vi "presentation_software.vi"() -> ()   [LabVIEW 2014]
uses:
  stateCtl.ctl
  <vilib>/Instr/_visa.llb/VISA Configure Serial Port (Instr).vi
panel:
  out "String":string
  in  "AnalogOutputDT":dbl(slide) scale=0.0..100.0
  out "Led1":bool
  in  "Output1":bool
  out "Led0":bool
  in  "Output0":bool
  out "S6":dbl
  out "S5":dbl
  out "S4":dbl
  out "S3":dbl
  out "S2":dbl
  out "S1":dbl
  out "S0":dbl
  in  "Tab Control":T1(tab)
  out "Frequency":dbl(graph)
  out "Temperature 1":dbl(graph)
  out "Temperature 2":dbl(graph)
  out "Load Cell 1":dbl(graph)
  out "Load Cell 2":dbl(graph)
  out "Vibration":dbl(graph)
  out "Analog Output":dbl(graph)
  out "exitLed":bool
  out "statusBar":string="     "
  in  "startButton":bool
  out "stopLed":bool
  out "startLed":bool
  in  "VISA Serial Port":refnum<visa-resource-name>
  in  "exitButton":bool
  in  "stopButton":bool
  out "FE":string
  out "FP":string
  out "isRunning":bool
  out "state":T2=enum."exit"
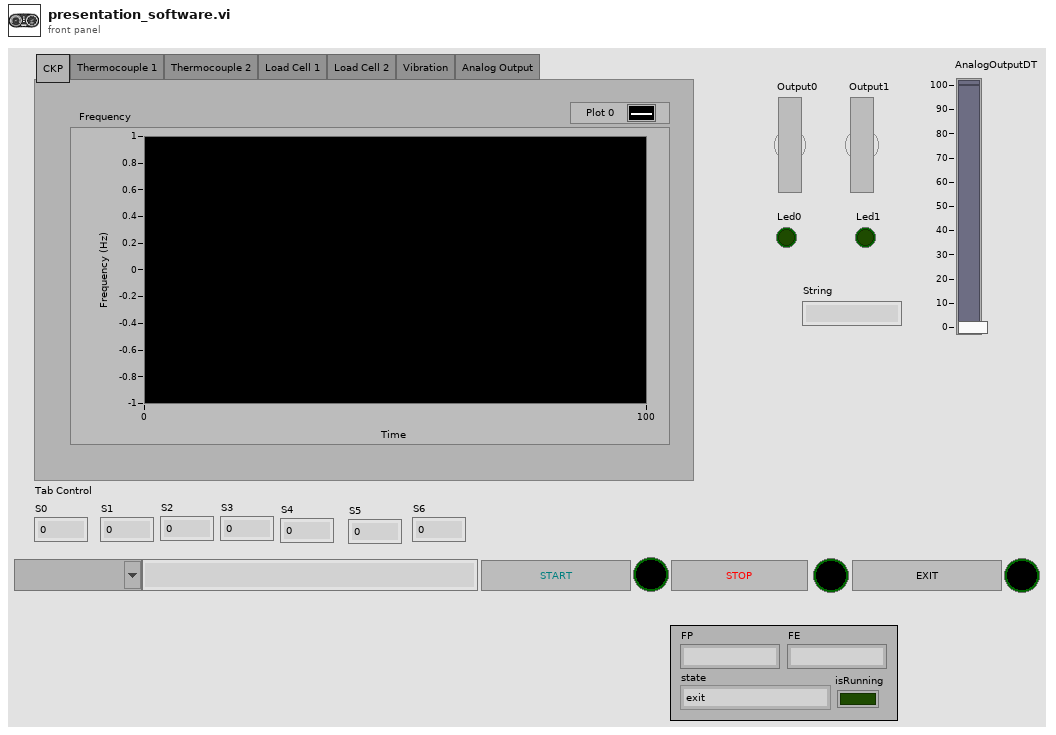
[diagram p1: front panel]
types:
  T1 = enum32{"CKP", "Thermocouple 1", "Thermocouple 2", "Load Cell 1", "Load Cell 2", "Vibration", "Analog Output"}
  T2 = typedef "stateCtl.ctl" = enum16{"init", "ready", "running", "stopped", "exit"}
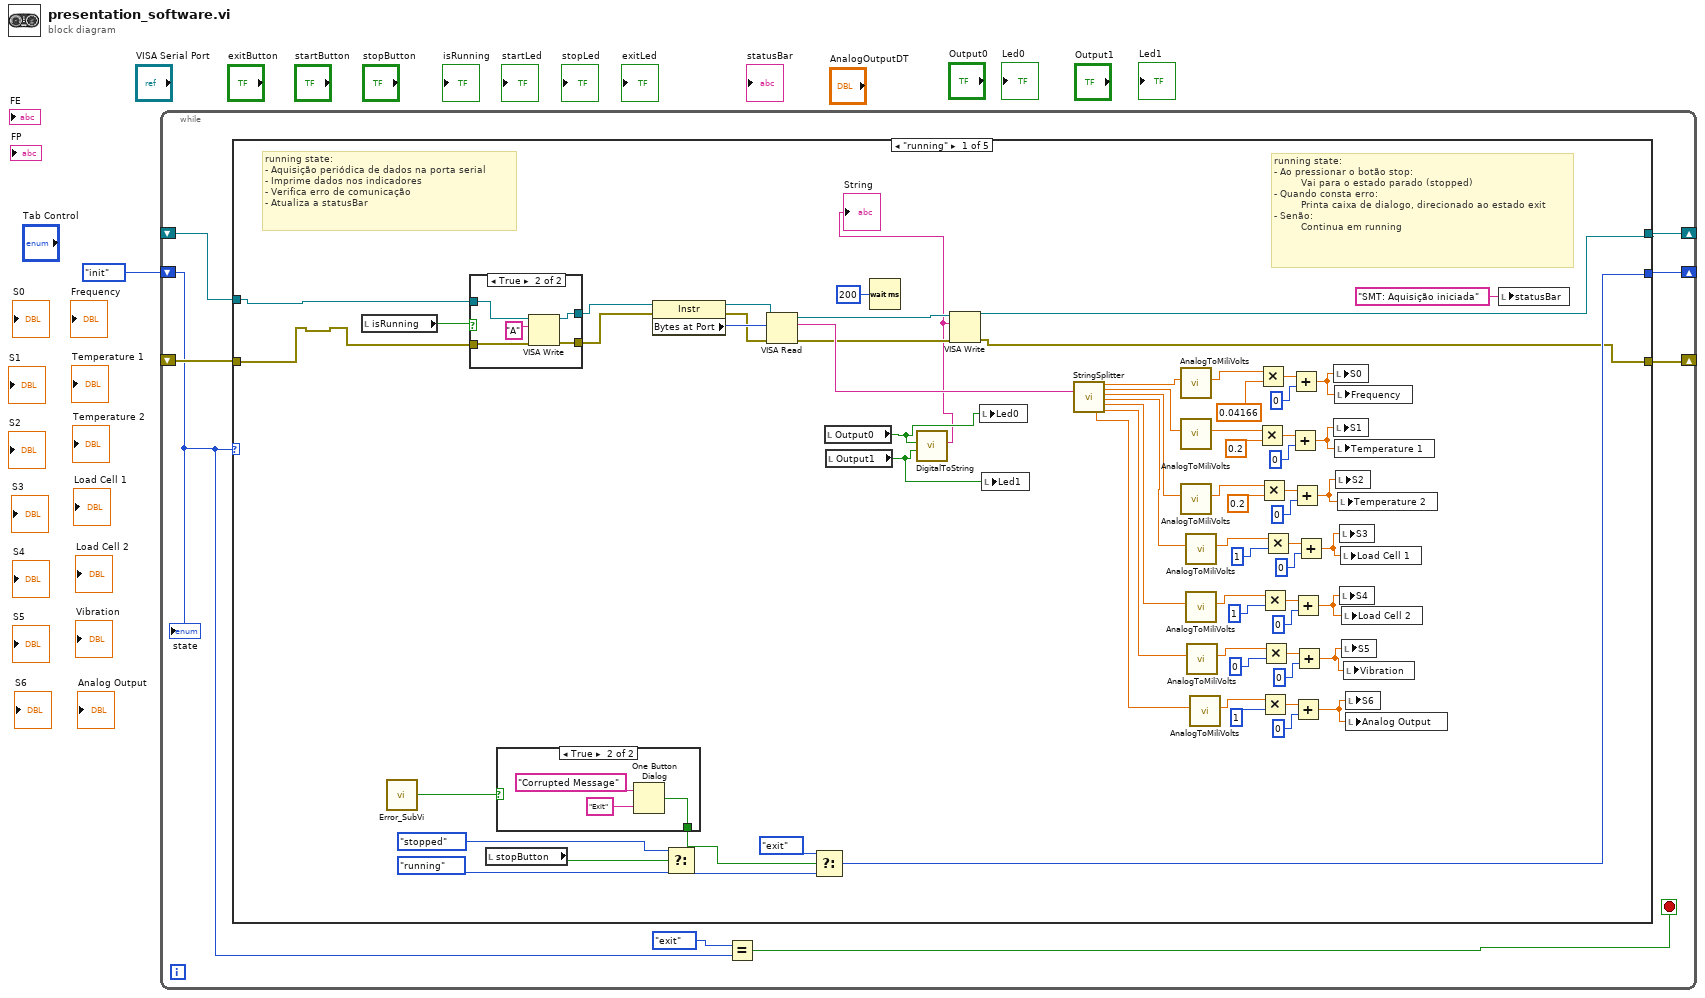
[diagram p0: block diagram]
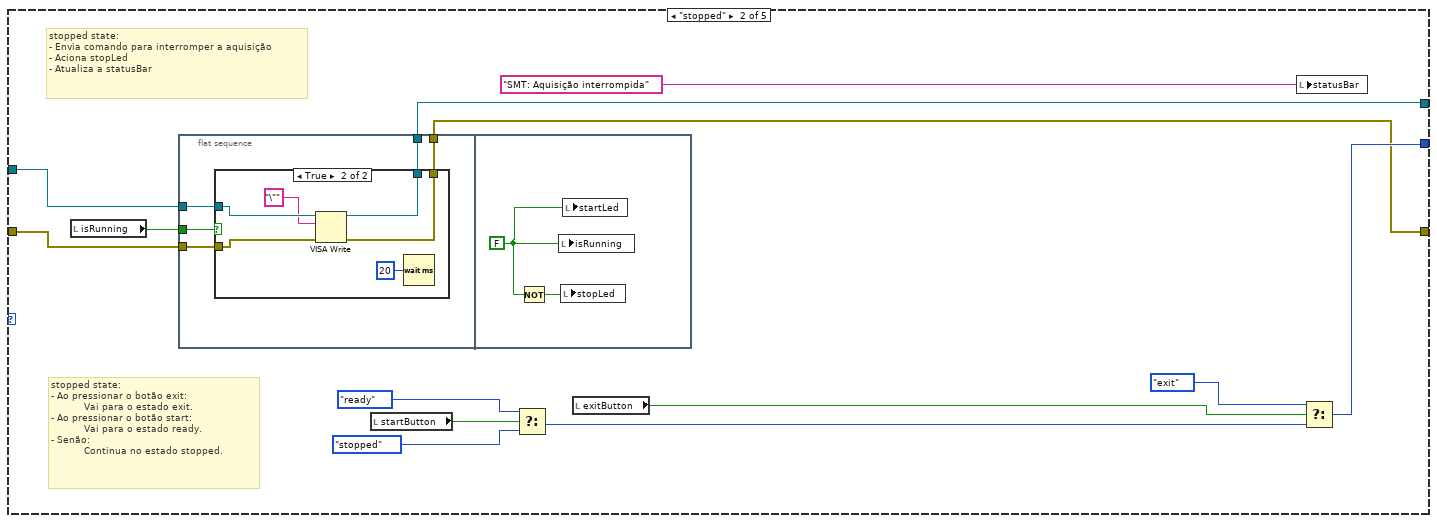
[diagram p4: hidden frame]
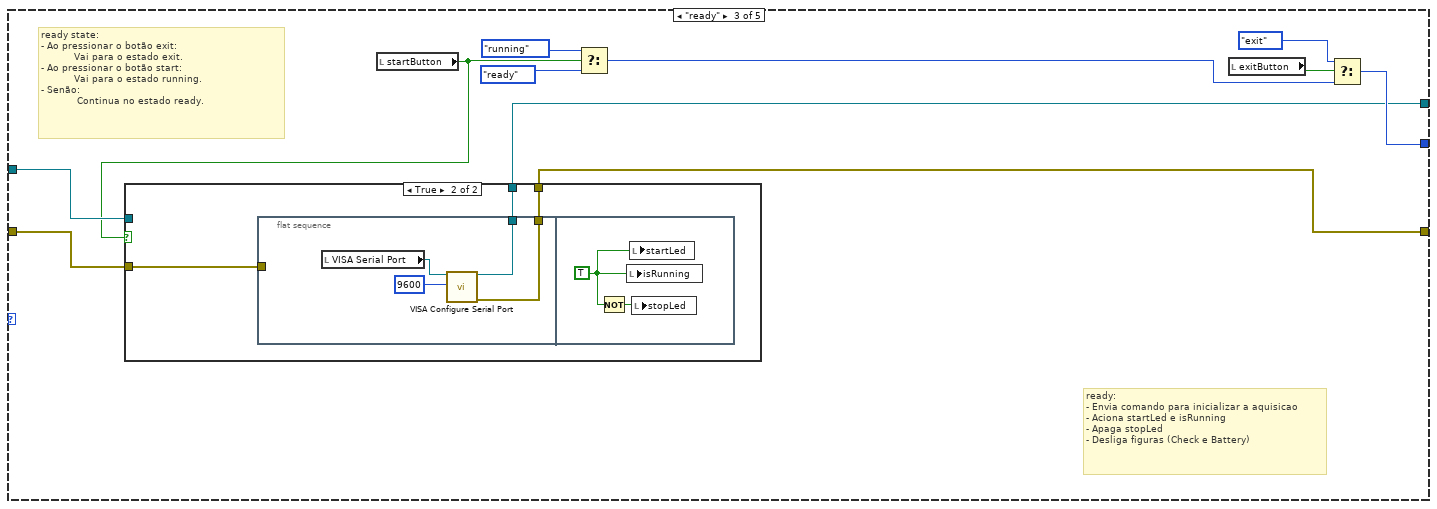
[diagram p6: hidden frame]
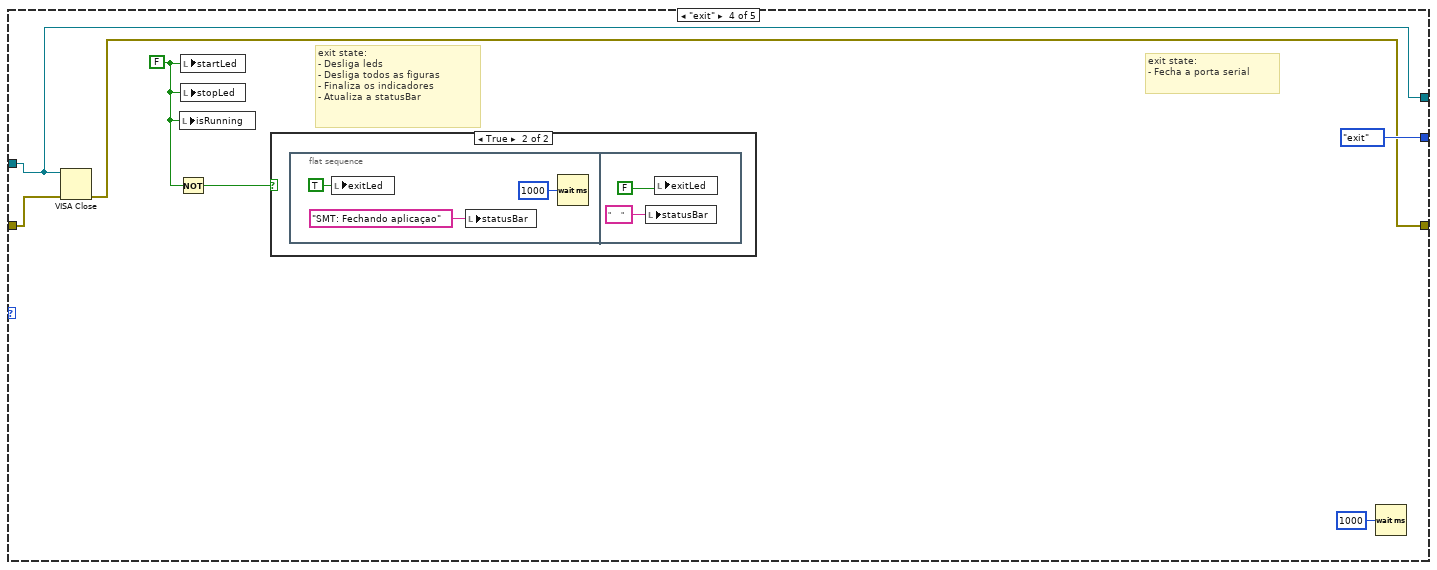
[diagram p8: hidden frame]
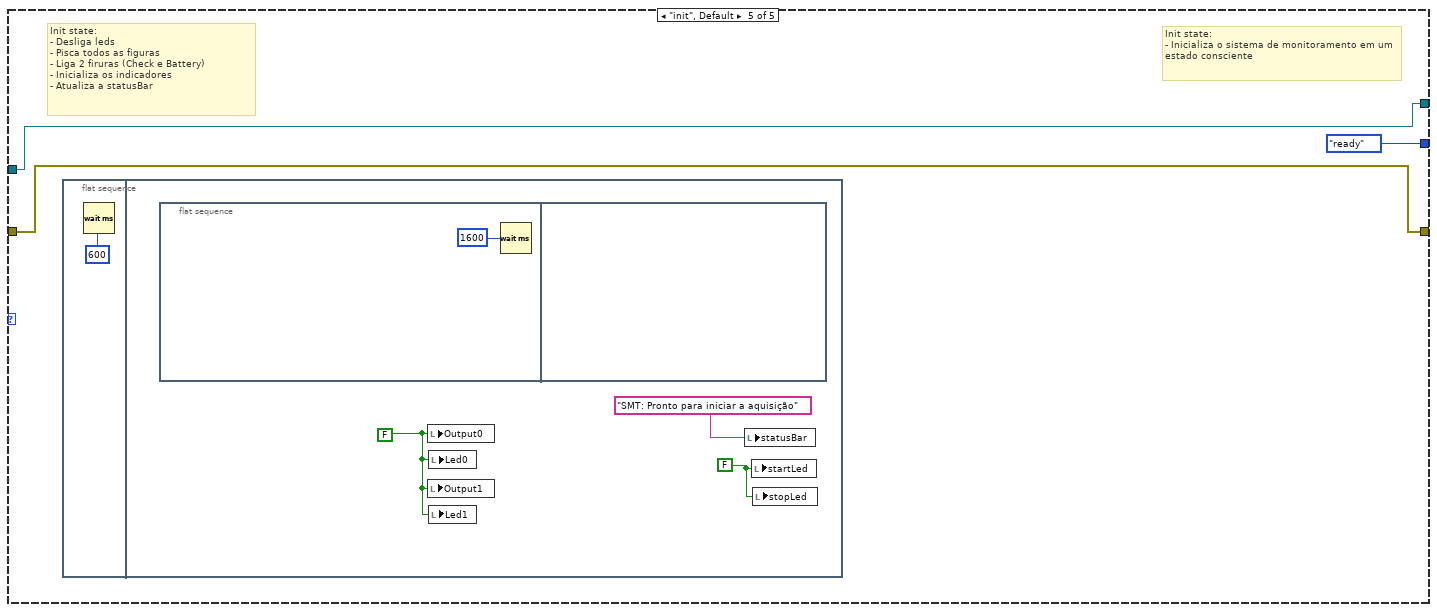
[diagram p10: hidden frame]
diagram:
  n1 = while {
    shift-right: [w3] -> _
    shift-left: _ -> [w8]
    shift-right: [w9] -> _
    shift-left: _ -> [w7]
    shift-right: [w4] -> _
    shift-left: stateCtl."init" ("state") -> [w5]
    stop <- w2 stop-if-true
    n2 = case shown="\"running\"" w5 {
      tunnel: [w16 w93 w119 w142 w152] -> w3
      tunnel: [w15 w94 w118 w143 w151] -> w9
      tunnel: [w66 w99 w122 stateCtl."exit" ("state") stateCtl."ready" ("state")] -> w4
      tunnel: w8 -> [w17 w97 w120 w142 w152]
      tunnel: w7 -> [w18 w96 w121 w144 w151]
      frame "running" {
        # "running state:\n- Ao pressionar o botão stop: \n         Vai para o estado parado (stopped)\n- Quando consta erro:\n         Printa caixa de dialogo, direcionado ao estado exit  \n- Senão:          \n         Continua em running"
        # "running state:\n- Aquisição periódica de dados na porta serial\n- Imprime dados nos indicadores\n- Verifica erro de comunicação\n- Atualiza a statusBar"
        n3 = local read "isRunning"() -> (w63:bool)
        n4 = call "Error_SubVi.vi"() -> ("error"=w62:bool)  [unwired: 11 in]
        n5 = case shown="True" w63 {
          tunnel: [w83 w87] -> w69
          tunnel: [w82 w86] -> w68
          tunnel: w18 -> [w83 w85]
          tunnel: w17 -> [w82 w84]
          frame False {
          }
          frame True {
            n6 = VISA Write(VISA resource name=w84, write buffer="A", error in (no error)=w85) -> (VISA resource name out=w86:refnum<visa-resource-name>, error out=w87:errorcluster)  [unwired: 1 out]
          }
        }
        n7 = local read "stopButton"() -> (w75:bool)
        n8 = case shown="True" w62 {
          selector: w62 -> [w78 _]
          tunnel: [w78 w79] -> w64
          frame False {
          }
          frame True {
            n9 = One Button Dialog(message="Corrupted Message", button name ("OK")="Exit") -> (true=w79:bool)
          }
        }
        n10 = property class="Instr"(reference=w68, error in=w69) -> (reference out=w71:refnum<visa-resource-name>, error out=w72:errorcluster, "Bytes at Port"=w73:u32)
        n11 = Select(t=stateCtl."stopped" ("state"), s=w75, f=stateCtl."running" ("state")) -> (s? t:f=w65:T2)
        n12 = VISA Read(VISA resource name=w71, byte count=w73, error in (no error)=w72) -> (VISA resource name out=w14:refnum<visa-resource-name>, read buffer=w19:string, error out=w13:errorcluster)  [unwired: 1 out]
        n13 = Select(t=stateCtl."exit" ("state"), s=w64, f=w65) -> (s? t:f=w66:T2)
        n14 = local read "Output0"() -> (w11:bool)
        n15 = local read "Output1"() -> (w12:bool)
        n16 = Wait (ms)(milliseconds to wait=u32 200) -> ()  [unwired: 1 out]
        n17 = call "DigitalToString.vi"("D1"=w12, "D0"=w11) -> ("Out"=w10:string)  [unwired: 9 in]
        "String" <- w10
        n18 = VISA Write(VISA resource name=w14, write buffer=w10, error in (no error)=w13) -> (VISA resource name out=w16:refnum<visa-resource-name>, error out=w15:errorcluster)  [unwired: 1 out]
        n19 = local write "Led0"(w11) -> ()
        n20 = local write "Led1"(w12) -> ()
        n21 = call "StringSplitter.vi"("Input String"=w19) -> ("S6"=w20:dbl, "S0"=w26:dbl, "S1"=w25:dbl, "S2"=w24:dbl, "S3"=w23:dbl, "S4"=w22:dbl, "S5"=w21:dbl)  [unwired: 11 in, 1 out]
        n22 = call "AnalogToMiliVolts.vi"("Input"=w26) -> ("Output"=w27:dbl)  [unwired: 10 in]
        n23 = call "AnalogToMiliVolts.vi"("Input"=w25) -> ("Output"=w28:dbl)  [unwired: 10 in]
        n24 = call "AnalogToMiliVolts.vi"("Input"=w24) -> ("Output"=w29:dbl)  [unwired: 10 in]
        n25 = call "AnalogToMiliVolts.vi"("Input"=w23) -> ("Output"=w30:dbl)  [unwired: 10 in]
        n26 = call "AnalogToMiliVolts.vi"("Input"=w22) -> ("Output"=w31:dbl)  [unwired: 10 in]
        n27 = call "AnalogToMiliVolts.vi"("Input"=w21) -> ("Output"=w32:dbl)  [unwired: 10 in]
        n28 = call "AnalogToMiliVolts.vi"("Input"=w20) -> ("Output"=w33:dbl)  [unwired: 10 in]
        n29 = Multiply(x=w28, y=0.2) -> (x*y=w57:dbl)
        n30 = Multiply(x=w27, y=0.04166) -> (x*y=w60:dbl)
        n31 = Multiply(x=w29, y=0.2) -> (x*y=w54:dbl)
        n32 = Multiply(x=w31, y=1) -> (x*y=w48:dbl)
        n33 = Multiply(x=w33, y=1) -> (x*y=w42:dbl)
        n34 = Multiply(x=w32, y=0) -> (x*y=w45:dbl)
        n35 = Multiply(x=w30, y=1) -> (x*y=w51:dbl)
        n36 = Add(x=w57, y=0) -> (x+y=w39:dbl)
        n37 = Add(x=w60, y=0) -> (x+y=w40:dbl)
        n38 = Add(x=w54, y=0) -> (x+y=w38:dbl)
        n39 = Add(x=w48, y=0) -> (x+y=w36:dbl)
        n40 = Add(x=w42, y=0) -> (x+y=w34:dbl)
        n41 = Add(x=w45, y=0) -> (x+y=w35:dbl)
        n42 = Add(x=w51, y=0) -> (x+y=w37:dbl)
        n43 = local write "S0"(w40) -> ()
        n44 = local write "S1"(w39) -> ()
        n45 = local write "Frequency"(w40) -> ()
        n46 = local write "Temperature 1"(w39) -> ()
        n47 = local write "S2"(w38) -> ()
        n48 = local write "Temperature 2"(w38) -> ()
        n49 = local write "S3"(w37) -> ()
        n50 = local write "S4"(w36) -> ()
        n51 = local write "Load Cell 1"(w37) -> ()
        n52 = local write "Load Cell 2"(w36) -> ()
        n53 = local write "S5"(w35) -> ()
        n54 = local write "Vibration"(w35) -> ()
        n55 = local write "S6"(w34) -> ()
        n56 = local write "Analog Output"(w34) -> ()
        n57 = local write "statusBar"("SMT: Aquisição iniciada" ("statusBar")) -> ()
      }
      frame "stopped" {
        # "stopped state:\n- Ao pressionar o botão exit: \n           Vai para o estado exit.\n- Ao pressionar o botão start:\n           Vai para o estado ready.\n- Senão:\n           Continua no estado stopped."
        # "stopped state:\n- Envia comando para interromper a aquisição\n- Aciona stopLed\n- Atualiza a statusBar"
        n58 = local read "isRunning"() -> (w95:bool)
        n59 = flat-sequence {
          tunnel: w97 -> [w106]
          tunnel: w96 -> [w105]
          tunnel: w95 -> [w104]
          tunnel: [w103] -> w94
          tunnel: [w102] -> w93
          frame #0 {
            n60 = case shown="True" w104 {
              tunnel: w106 -> [w108 w114]
              tunnel: w105 -> [w107 w113]
              tunnel: [w107 w109] -> w103
              tunnel: [w108 w111] -> w102
              frame False {
              }
              frame True {
                n61 = VISA Write(VISA resource name=w114, write buffer="\"", error in (no error)=w113) -> (VISA resource name out=w111:refnum<visa-resource-name>, error out=w109:errorcluster)  [unwired: 1 out]
                n62 = Wait (ms)(milliseconds to wait=u32 20) -> ()  [unwired: 1 out]
              }
            }
          }
          frame #1 {
            w116 = FALSE ("Boolean")
            n63 = Not(x=w116) -> (.not. x?=w115:bool)
            n64 = local write "isRunning"(w116) -> ()
            n65 = local write "stopLed"(w115) -> ()
            n66 = local write "startLed"(w116) -> ()
          }
        }
        n67 = local read "startButton"() -> (w92:bool)
        n68 = Select(t=stateCtl."ready" ("state"), s=w92, f=stateCtl."stopped" ("state")) -> (s? t:f=w100:T2)
        n69 = local read "exitButton"() -> (w91:bool)
        n70 = local write "statusBar"("SMT: Aquisição interrompida" ("statusBar")) -> ()
        n71 = Select(t=stateCtl."exit" ("state"), s=w91, f=w100) -> (s? t:f=w99:T2)
      }
      frame "ready" {
        # "ready state:\n- Ao pressionar o botão exit: \n           Vai para o estado exit.\n- Ao pressionar o botão start:\n           Vai para o estado running.\n- Senão:\n            Continua no estado ready."
        # "ready:\n- Envia comando para inicializar a aquisicao\n- Aciona startLed e isRunning\n- Apaga stopLed\n- Desliga figuras (Check e Battery)"
        n72 = local read "startButton"() -> (w117:bool)
        n73 = case shown="True" w117 {
          tunnel: [w129 w130] -> w119
          tunnel: [w128 w131] -> w118
          tunnel: w120 -> [w129 _]
          tunnel: w121 -> [w128 w132]
          frame False {
          }
          frame True {
            n74 = flat-sequence {
              tunnel: w132 -> [_]
              tunnel: [w134] -> w131
              tunnel: [w133] -> w130
              frame #0 {
                n75 = local read "VISA Serial Port"() -> (w135:refnum<visa-resource-name>)
                n76 = call-poly "VISA Configure Serial Port"("VISA resource name"=w135, "baud rate (9600)"=u32 9600) -> ("VISA resource name out"=w133:refnum<visa-resource-name>, "error out"=w134:errorcluster)  [unwired: 12 in]
              }
              frame #1 {
                w138 = TRUE ("Boolean")
                n77 = Not(x=w138) -> (.not. x?=w137:bool)
                n78 = local write "isRunning"(w138) -> ()
                n79 = local write "startLed"(w138) -> ()
                n80 = local write "stopLed"(w137) -> ()
              }
            }
          }
        }
        n81 = Select(t=stateCtl."running" ("state"), s=w117, f=stateCtl."ready" ("state")) -> (s? t:f=w123:T2)
        n82 = local read "exitButton"() -> (w125:bool)
        n83 = Select(t=stateCtl."exit" ("state"), s=w125, f=w123) -> (s? t:f=w122:T2)
      }
      frame "exit" {
        w140 = FALSE ("startLed")
        # "exit state:\n- Desliga leds\n- Desliga todos as figuras\n- Finaliza os indicadores\n- Atualiza a statusBar"
        # "exit state:\n- Fecha a porta serial"
        n84 = VISA Close(VISA resource name=w142, error in (no error)=w144) -> (error out=w143:errorcluster)
        n85 = Not(x=w140) -> (.not. x?=w141:bool)
        n86 = local write "isRunning"(w140) -> ()
        n87 = local write "startLed"(w140) -> ()
        n88 = local write "stopLed"(w140) -> ()
        n89 = case shown="True" w141 {
          frame False {
          }
          frame True {
            n90 = flat-sequence {
              frame #0 {
                n91 = local write "exitLed"(TRUE ("exitLed")) -> ()
                n92 = local write "statusBar"("SMT: Fechando aplicaçao" ("statusBar")) -> ()
                n93 = Wait (ms)(milliseconds to wait=u32 1000) -> ()  [unwired: 1 out]
              }
              frame #1 {
                n94 = local write "statusBar"("     " ("statusBar")) -> ()
                n95 = local write "exitLed"(FALSE ("exitLed")) -> ()
              }
            }
          }
        }
        n96 = Wait (ms)(milliseconds to wait=u32 1000) -> ()  [unwired: 1 out]
      }
      frame "init", Default {
        # "Init state:\n- Inicializa o sistema de monitoramento em um estado consciente"
        # "Init state:\n- Desliga leds\n- Pisca todos as figuras\n- Liga 2 firuras (Check e Battery)\n- Inicializa os indicadores\n- Atualiza a statusBar"
        n97 = flat-sequence {
          frame #0 {
            n98 = Wait (ms)(milliseconds to wait=u32 600) -> ()  [unwired: 1 out]
          }
          frame #1 {
            w155 = FALSE
            w157 = FALSE
            n99 = flat-sequence {
              frame #0 {
                n100 = Wait (ms)(milliseconds to wait=u32 1600) -> ()  [unwired: 1 out]
              }
              frame #1 {
              }
            }
            n101 = local write "Output0"(w155) -> ()
            n102 = local write "Output1"(w155) -> ()
            n103 = local write "Led0"(w155) -> ()
            n104 = local write "Led1"(w155) -> ()
            n105 = local write "statusBar"("SMT: Pronto para iniciar a aquisição" ("statusBar")) -> ()
            n106 = local write "startLed"(w157) -> ()
            n107 = local write "stopLed"(w157) -> ()
          }
        }
      }
    }
    n108 = Equal?(x=stateCtl."exit" ("state"), y=w5) -> (x = y?=w2:bool)
    "state" <- w5
  }
